vi "Check for an existing project.vi"(0 "Base folder":path, 7 "Project name":string, 11 "error in":errorcluster) -> (3 "Comment":string, 4 "Project folder":path, 6 "ini file path":path, 8 "data":T1, 10 "Project exists":bool, 13 "Project folder exists":bool, 14 "Project ini exists":bool, 15 "error out":errorcluster)   [LabVIEW 2011]
uses:
  Project in icluster.ctl
  GUI/Job setup/Job and site cluster.ctl
  emi cndiates/List of all contrys(combo box).ctl
  GUI/Job setup/Tool registration ID.ctl
  Run Information.ctl
  <vilib>/Utility/VariantDataType/VariantType.lvlib
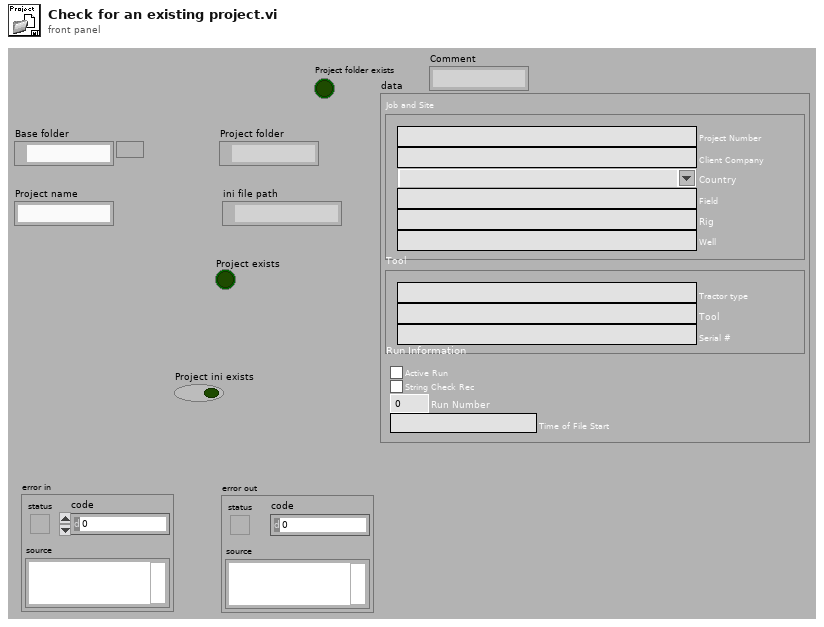
[diagram p1: front panel]
types:
  T1 = typedef "Project in icluster.ctl" = cluster{"Job and Site":T2, "Tool":T4, "Run Information":T5}
  T2 = typedef "Job and site cluster.ctl" = cluster{"Project Number":string, "Client Company":string, "Country":T3, "Field":string, "Rig":string, "Well":string}
  T3 = typedef "List of all contrys(combo box).ctl" = string
  T4 = typedef "Tool registration ID.ctl" = cluster{"Tractor type":string, "Tool":string, "Serial #":string}
  T5 = typedef "Run Information.ctl" = cluster{"Active Run":bool, "String Check Rec":bool, "Run Number":i32, "Time of File Start":string}
  T6 = enum16{"open", "replace", "create", "open or create", "replace or create", "replace or create with confirmation"}
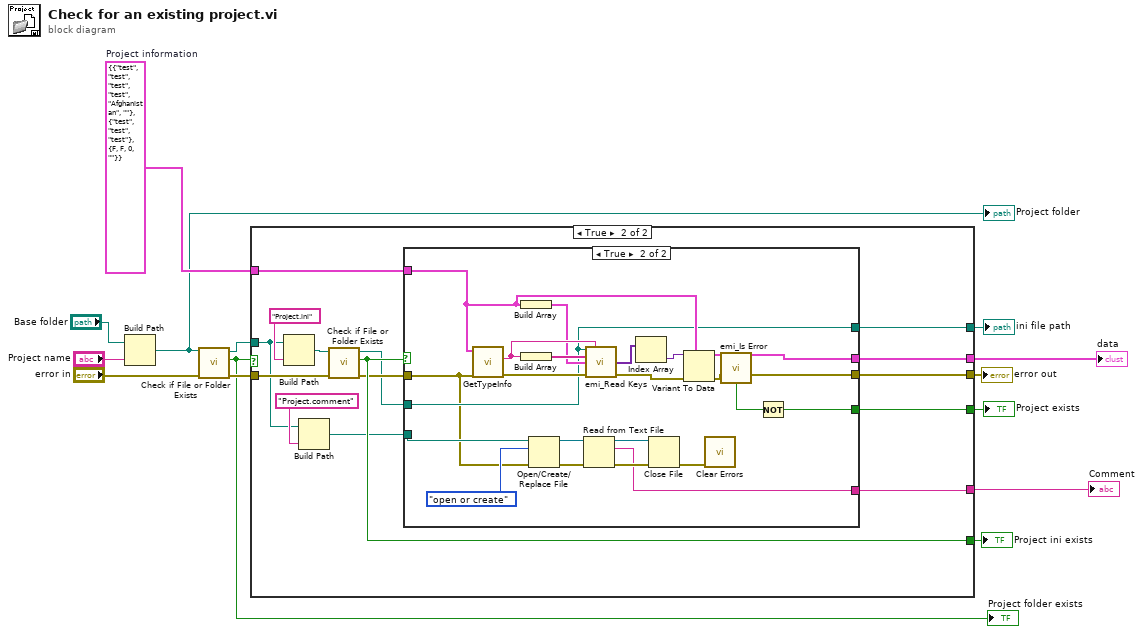
[diagram p0: block diagram]
diagram:
  w11 = T1 {"Job and Site"={"Project Number"="test", "Client Company"="test", "Country"="test", "Field"="test", "Rig"="Afghanistan", "Well"=""}, "Tool"={"Tractor type"="test", "Tool"="test", "Serial #"="test"}, "Run Information"={"Active Run"=FALSE, "String Check Rec"=FALSE, "Run Number"=0, "Time of File Start"=""}}  # Project information
  n1 = Build Path(base path="Base folder", name or relative path="Project name") -> (appended path=w4:path)
  "Project folder" <- w4
  n2 = call <vilib>:"Check if File or Folder Exists.vi"("error in (no error)"="error in", "path"=w4) -> ("error out"=w5:errorcluster, "file or folder exists?"=w2:bool, "dup path"=w3:path)  [unwired: 7 in]
  "Project folder exists" <- w2
  n3 = case shown="True" w2 {
    tunnel: w3 -> [w15 w19]
    tunnel: [_ w29] -> w12
    tunnel: w11 -> [_ w27]
    tunnel: [_ w25] -> w10
    tunnel: [w16 w24] -> w9
    tunnel: [_ w23] -> w8
    tunnel: [w15 w22] -> w7
    tunnel: w5 -> [w16 w21]
    tunnel: [_ w17] -> w1
    frame False {
    }
    frame True {
      n4 = Build Path(base path=w19, name or relative path="Project.ini") -> (appended path=w31:path)
      n5 = Build Path(base path=w19, name or relative path="Project.comment") -> (appended path=w18:path)
      n6 = call <vilib>:"Check if File or Folder Exists.vi"("error in (no error)"=w21, "path"=w31) -> ("error out"=w28:errorcluster, "file or folder exists?"=w29:bool, "dup path"=w26:path)  [unwired: 7 in]
      n7 = case shown="True" w29 {
        tunnel: w28 -> [w33 w40]
        tunnel: w27 -> [_ w49]
        tunnel: w26 -> [w32 w43]
        tunnel: [_ w48] -> w25
        tunnel: [w33 w44] -> w24
        tunnel: [_ w45] -> w23
        tunnel: [w32 w43] -> w22
        tunnel: w18 -> [_ w42]
        tunnel: [_ w34] -> w17
        frame False {
        }
        frame True {
          n8 = call <vilib>:"GetTypeInfo.vi"("error in (no error)"=w40, "Variant"=w49) -> ("error out"=w51:errorcluster, "Name"=w53:string)  [unwired: 5 in, 3 out]
          n9 = Build Array(w49) -> (w50:T1[])
          n10 = Build Array(w53) -> (w52:string[])
          n11 = Open/Create/Replace File(file path (use dialog)=w42, error in=w40, operation (0:open)=T6."open or create") -> (refnum out=w38:refnum<file>, error out=w39:errorcluster)  [unwired: 3 in, 1 out]
          n12 = Read from Text File(file (use dialog)=w38, error in=w39) -> (refnum out=w36:refnum<file>, text=w34:string, error out=w37:errorcluster)  [unwired: 2 in, 1 out]
          n13 = call "emi_Read Keys.vi"("Ini Path(..app../config.ini)"=w43, "Section"=w53, "Key Names"=w52, "Types/Defaults"=w50, "error in (no error)"=w51) -> ("Values"=w54:variant[], "error out"=w55:errorcluster)  [unwired: 8 in, 1 out]
          n14 = Index Array(array=w54) -> (element=w56:variant)  [unwired: 1 in]
          n15 = Close File(refnum=w36, error in=w37) -> (error out=w35:errorcluster)  [unwired: 1 out]
          n16 = Variant To Data(error in=w55, type=w49, Variant=w56) -> (data=w48:T1, error out=w47:errorcluster)
          n17 = call <vilib>:"Clear Errors.vi"("error in (no error)"=w35) -> ()  [unwired: 6 in, 1 out]
          n18 = call "emi_Is Error.vi"("error in (no error)"=w47) -> ("error out"=w44:errorcluster, "Is Error"=w46:bool)  [unwired: 13 in]
          n19 = Not(x=w46) -> (.not. x?=w45:bool)
        }
      }
    }
  }
  "error out" <- w9
  "ini file path" <- w7
  "Project ini exists" <- w12
  "data" <- w10
  "Project exists" <- w8
  "Comment" <- w1
